vi "CommonTrigger.vi"(8 "error in (no error)":errorcluster, 10 "MasterTriggerCounter":i64, 11 "BME_DG_Base in":refnum<class "BME_DG_Base.lvclass">) -> (0 "error out":errorcluster, 1 "CountsTillCommonTrg":i64, 2 "TriggerModuloLCMult":i64, 3 "BME_DG_Base out":refnum<class "BME_DG_Base.lvclass">)   [LabVIEW 2009, in "POLARIS BME DG.lvlib" / "BME_DG_Base.lvclass"]
uses:
  BME_DG_Base.lvclass
  BME_DG_Base.lvclass/BME_DG_Base.ctl
  BME_DG_Chnl/BME_DG_Chnl.lvclass
  POLARIS BME DG.lvlib
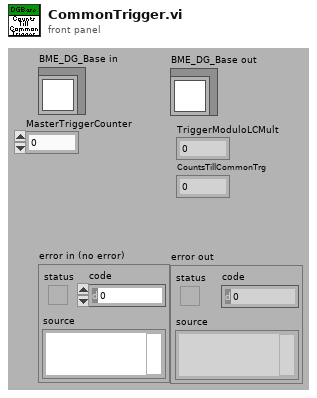
[diagram p1: front panel]
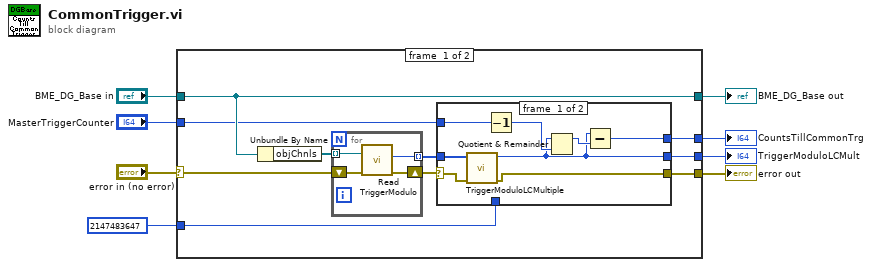
[diagram p0: block diagram]
diagram:
  n1 = case shown="No Error" "error in (no error)" {
    selector: "error in (no error)" -> [w12 w34]
    tunnel: [w11 w34] -> w7
    tunnel: [w18 w33] -> w5
    tunnel: "BME_DG_Base in" -> [w18 w33]
    tunnel: [w14 w32] -> w3
    tunnel: 2147483647 ("LeastCommonMult") -> [w13 w32]
    tunnel: [w10 w32] -> w2
    tunnel: "MasterTriggerCounter" -> [w9 _]
    frame #0 {
      n2 = Unbundle By Name(w18) -> ("objChnls"=w17:refnum<class "BME_DG_Chnl.lvclass">[])
      n3 = for {
        tunnel: w17 -> [w31] mode=indexing
        tunnel: [w29] -> w16 mode=indexing
        shift-right: [w28] -> w15
        shift-left: w12 -> [w30]
        n4 = call-dynamic "Read TriggerModulo.vi"("error in (no error)"=w30, "BME_DG_Chnl in"=w31) -> ("error out"=w28:errorcluster, "TriggerModulo"=w29:i32)  [unwired: 7 in, 1 out]
      }
      n5 = case shown="No Error" w15 {
        selector: w15 -> [w24 w27]
        tunnel: w16 -> [w25 _]
        tunnel: [w19 w26] -> w14
        tunnel: w13 -> [_ w26]
        tunnel: [w24 w27] -> w11
        tunnel: w9 -> [w23 _]
        tunnel: [w20 w26] -> w10
        frame #0 {
          n6 = call "TriggerModuloLCMultiple.vi"("TriggerModulos"=w25) -> ("LeastCommonMult"=w19:i64)  [unwired: 10 in]
          n7 = Decrement(x=w23) -> (x-1=w21:i64)
          n8 = Quotient & Remainder(x=w19, y=w21) -> (x-y*floor(x/y)=w22:i64)  [unwired: 1 out]
          n9 = Subtract(x=w19, y=w22) -> (x-y=w20:i64)
        }
        frame #1 {
        }
      }
    }
    frame #1 {
    }
  }
  "error out" <- w7
  "BME_DG_Base out" <- w5
  "TriggerModuloLCMult" <- w3
  "CountsTillCommonTrg" <- w2
